vi "Engine-RPC.vi"(8 "Error In":errorcluster, 11 "DSI Reference":refnum<class "DCM-DSI.lvclass">) -> (0 "Error Out":errorcluster, 3 "DSI Reference":refnum<class "DCM-DSI.lvclass">)   [LabVIEW 2016, in "DSI-RT.lvlib"]
uses:
  DSI-RT.lvlib
  Classes/DCM-DSI/DCM-DSI.lvclass
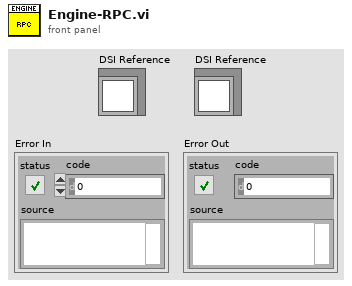
[diagram p1: front panel]
types:
  T1 = typedef "DSI-Shared.lvlib/Engine-RPC-Modes.ctl" = enum8{"Disabled", "DSI - PWM Pumps", "DSI - Sync Pumps"}
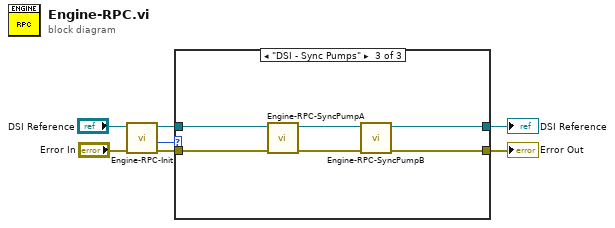
[diagram p0: block diagram]
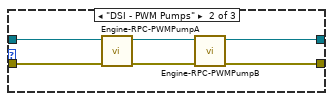
[diagram p3: hidden frame]
diagram:
  n1 = call "Engine-RPC-Init.vi"("Error In"="Error In", "DSI Reference"="DSI Reference") -> ("Error Out"=w4:errorcluster, "Control Mode"=w3:T1, "DSI Reference"=w5:refnum<class "DCM-DSI.lvclass">)  [unwired: 7 in]
  n2 = case shown="\"DSI - Sync Pumps\"" w3 {
    tunnel: [w8 w12 w18] -> w2
    tunnel: [w9 w10 w16] -> w1
    tunnel: w5 -> [w8 w15 w20]
    tunnel: w4 -> [w9 w14 w21]
    frame "Disabled", Default {
    }
    frame "DSI - PWM Pumps" {
      n3 = call "Engine-RPC-PWMPumpA.vi"("Error In"=w14, "DSI Reference"=w15) -> ("Error Out"=w11:errorcluster, "DSI Reference"=w13:refnum<class "DCM-DSI.lvclass">)  [unwired: 8 in]
      n4 = call "Engine-RPC-PWMPumpB.vi"("Error In"=w11, "DSI Reference"=w13) -> ("Error Out"=w10:errorcluster, "DSI Reference"=w12:refnum<class "DCM-DSI.lvclass">)  [unwired: 8 in]
    }
    frame "DSI - Sync Pumps" {
      n5 = call "Engine-RPC-SyncPumpA.vi"("Error In"=w21, "DSI Reference"=w20) -> ("Error Out"=w17:errorcluster, "DSI Reference"=w19:refnum<class "DCM-DSI.lvclass">)  [unwired: 8 in]
      n6 = call "Engine-RPC-SyncPumpB.vi"("Error In"=w17, "DSI Reference"=w19) -> ("Error Out"=w16:errorcluster, "DSI Reference"=w18:refnum<class "DCM-DSI.lvclass">)  [unwired: 8 in]
    }
  }
  "Error Out" <- w1
  "DSI Reference" <- w2
